vi "Untitled 2 (SubVI).vi"(0 "classes per student":i32, 4 "periods per day":i32, 5 "number of students":i32, 6 "error out":errorcluster, 7 "min class size":i32, 8 "max class size":i32) -> (1 "progress":i32(slide) scale=0.01..95.0, 2 "Array":dbl[][](array[numeric]), 3 "number of class courses":i32)   [LabVIEW 2009]
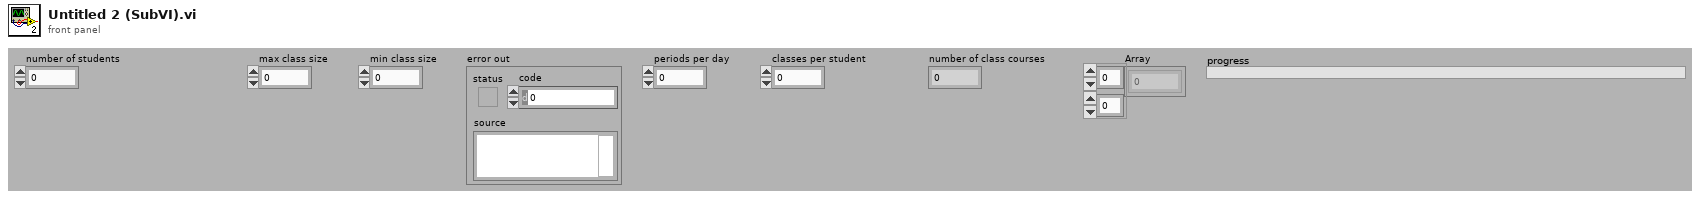
[diagram p1: front panel]
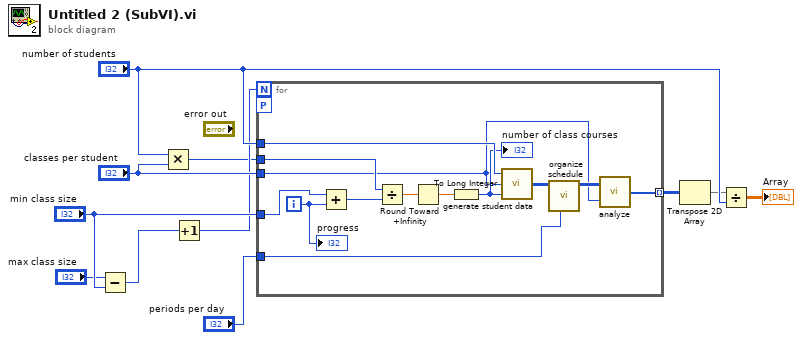
[diagram p0: block diagram]
diagram:
  n1 = Subtract(x="max class size", y="min class size") -> (x-y=w5:i32)
  n2 = Multiply(x="number of students", y="classes per student") -> (x*y=w1:i32)
  n3 = Increment(x=w5) -> (x+1=w4:i32)
  n4 = for {
    N: w4 -> [_]
    tunnel: "classes per student" -> [w14]
    tunnel: "number of students" -> [w22]
    tunnel: w1 -> [w21]
    tunnel: [w13] -> w2 mode=indexing
    tunnel: "min class size" -> [w17]
    workers-P: _ -> [_]
    tunnel: "periods per day" -> [w12]
    i -> [w18]
    n5 = Add(x=w17, y=w18) -> (x+y=w16:i32)
    n6 = Divide(x=w21, y=w16) -> (x/y=w20:dbl)
    n7 = Round Toward +Infinity(x=w20) -> (ceil(x): smallest int >= x=w15:dbl)
    n8 = To Long Integer(number=w15) -> (32bit integer=w19:i32)
    "number of class courses" <- w19
    n9 = call "generate student data.vi"("number of class courses"=w19, "classes per student"=w14, "number of students"=w22) -> ("Student data"=w24:i32[][])
    n10 = call "organize schedule.vi"("periods per day"=w12, "Student data"=w24) -> ("rearranged Student data"=w23:i32[][])  [unwired: 9 in]
    n11 = call "analyze.vi"("classes per student"=w14, "rearranged Student data"=w23) -> ("Array"=w13:i32[])
    "progress" <- w18
  }
  n12 = Transpose 2D Array(2D array=w2) -> (transposed array=w7:i32[][])
  n13 = Divide(x=w7, y="number of students") -> (x/y=→"Array":dbl[][])
